vi "ITR HP.vi"(7 "input":dbl format="%.2f", 13 "corner period (steps)":dbl(slide)=10.237739663395852 scale=1.0..1000.0) -> (8 "output":dbl format="%.2f")   [LabVIEW 2016]
doc: "Modular ITR first order high pass filter with internal shift registers.\n\nAlexis Lopez\nP350\nCSUSB Physics"
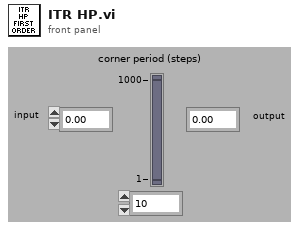
[diagram p1: front panel]
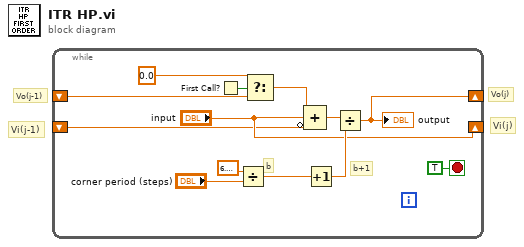
[diagram p0: block diagram]
diagram:
  # "Vi(j-1)"
  # "Vi(j)"
  # "Vo(j-1)"
  # "Vo(j)"
  n1 = while {
    shift-left: _ -> [w6]
    shift-right: [w8] -> _
    shift-right: ["input"] -> _
    shift-left: _ -> [w2]
    stop <- TRUE stop-if-true
    # "b+1"
    # "b"
    n2 = First Call?() -> (First Call?: T/F=w7:bool)
    n3 = Divide(x=6.283185307179586, y="corner period (steps)") -> (x/y=w10:dbl)
    n4 = Select(t=0.0, s=w7, f=w6) -> (s? t:f=w4:dbl)
    n5 = Compound Arithmetic op=ADD(w4, "input", invert w2) -> (w1:dbl)
    n6 = Increment(x=w10) -> (x+1=w9:dbl)
    n7 = Divide(x=w1, y=w9) -> (x/y=w8:dbl)
    "output" <- w8
  }
